vi "sort standard to sequence.vi"(8 "error in":errorcluster) -> (3 "output cluster":T1, 11 "cycle results cluster IN":T2)   [LabVIEW 2016]
doc: "Takes a sample type and sorts by sequence"
uses:
  controls/cycle results control.ctl
  controls/data control cluster.ctl
panel:
  out "Array":dbl[][][](array[numeric])
  out "error out":errorcluster
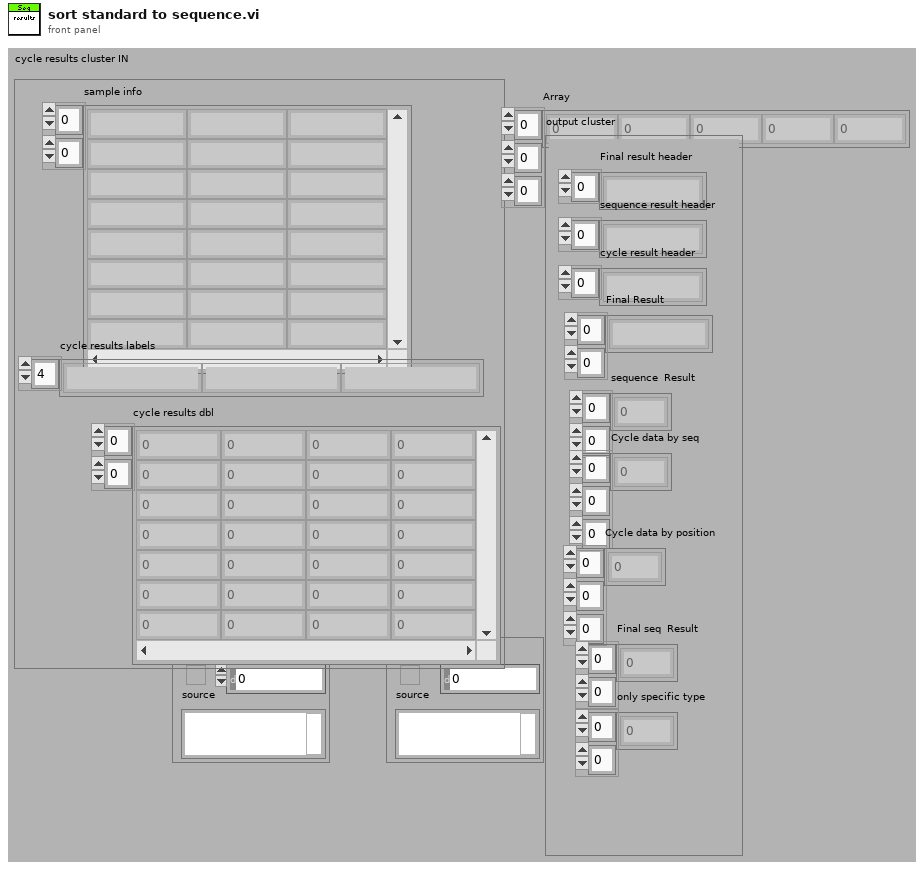
[diagram p1: front panel]
types:
  T1 = typedef "data control cluster.ctl" = cluster{"Final result header":string[], "sequence result header":string[], "cycle result header ":string[], "Final Result":string[][], "sequence  Result":dbl[][], "Cycle data by seq":dbl[][][], "Cycle data by position":dbl[][][], "Final seq  Result":dbl[][], "only specific type":dbl[][]}
  T2 = typedef "cycle results control.ctl" = cluster{"sample info":string[][], "cycle results labels":string[], "cycle results dbl":dbl[][]}
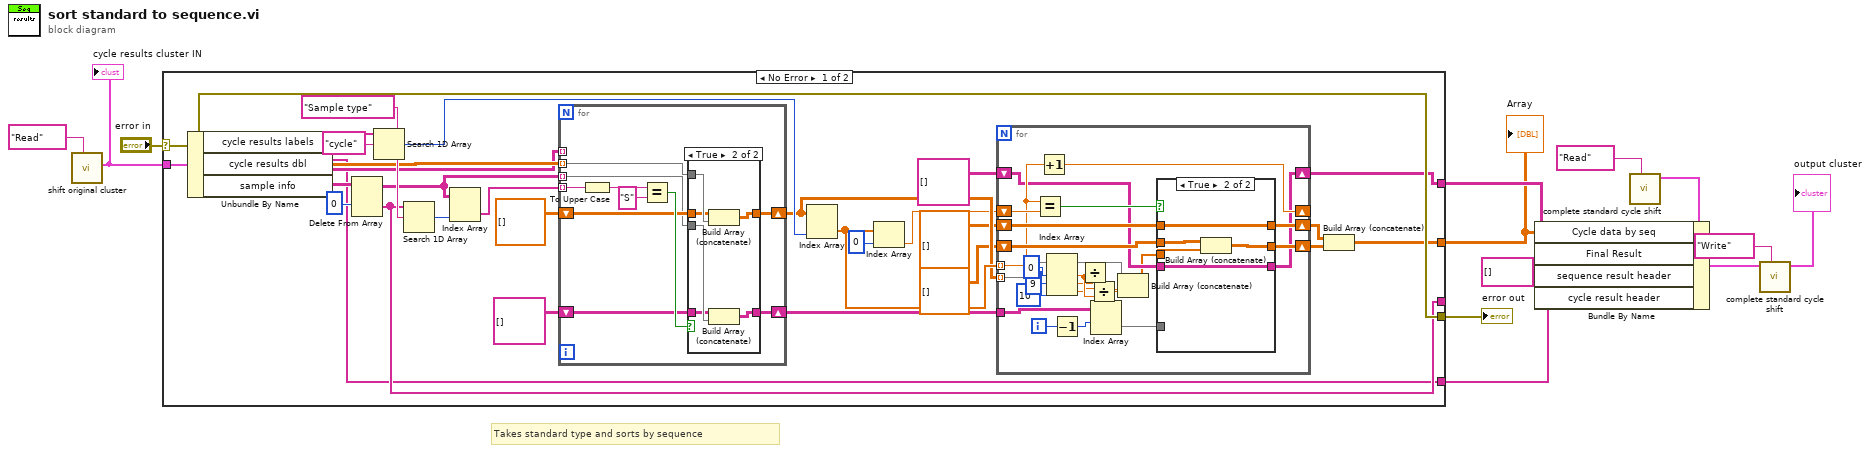
[diagram p0: block diagram]
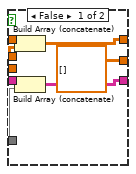
[diagram p2: hidden frame]
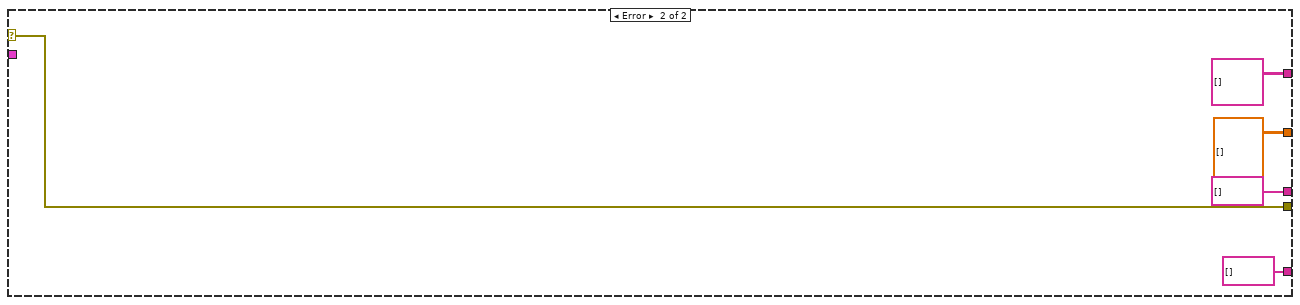
[diagram p4: hidden frame]
diagram:
  # "Takes standard type and sorts by sequence"
  n1 = call "shift original cluster.vi"("read write shift"="Read") -> ("cycle results cluster out"=w9:T2)  [unwired: 9 in, 1 out]
  "cycle results cluster IN" <- w9
  n2 = case shown="No Error" "error in" {
    selector: "error in" -> [w39 w98]
    tunnel: w9 -> [w38 _]
    tunnel: [w39 w98] -> w11
    tunnel: [w16 string[][] []] -> w5
    tunnel: [w15 string[] [] ("sample info")] -> _
    tunnel: [w14 dbl[][][] []] -> w4
    tunnel: [w13 string[] [] ("cycle results labels")] -> w1
    frame No Error {
      n3 = Unbundle By Name(w38) -> ("cycle results labels"=w13:string[], "cycle results dbl"=w33:dbl[][], "sample info"=w31:string[][])
      n4 = Delete From Array(array=w31, index (row)=0) -> (deleted portion=w15:string[], array with subset deleted=w30:string[][])  [unwired: 2 in]
      n5 = Search 1D Array(1D array=w13, element="cycle") -> (index of element=w27:i32)  [unwired: 1 in]
      n6 = Search 1D Array(1D array=w15, element="Sample type") -> (index of element=w35:i32)  [unwired: 1 in]
      n7 = Index Array(array=w30, index (col)=w35) -> (element=w34:string[])  [unwired: 1 in]
      n8 = for {
        tunnel: w31 -> [_] mode=indexing
        tunnel: w33 -> [w81] mode=indexing
        tunnel: w34 -> [w85] mode=indexing
        shift-right: [w80] -> w25
        shift-left: dbl[][] [] -> [w79]
        tunnel: w30 -> [w78] mode=indexing
        shift-right: [w77] -> w18
        shift-left: string[][] [] -> [w76]
        n9 = To Upper Case(1:w85) -> (0:w84:string)
        n10 = Equal?(x=w84, y="S") -> (x = y?=w82:bool)
        n11 = case shown="True" w82 {
          tunnel: w81 -> [_ w93]
          tunnel: [w87 w92] -> w80
          tunnel: w79 -> [w87 w91]
          tunnel: w78 -> [_ w90]
          tunnel: [w86 w88] -> w77
          tunnel: w76 -> [w86 w89]
          frame False {
          }
          frame True {
            n12 = Build Array (concatenate)(w91, w93) -> (w92:dbl[][])
            n13 = Build Array (concatenate)(w89, w90) -> (w88:string[][])
          }
        }
      }
      n14 = Index Array(array=w25, index (col)=w27) -> (element=w26:dbl[])  [unwired: 1 in]
      n15 = Index Array(array=w26, index=0) -> (element=w19:dbl)
      n16 = for {
        tunnel: w26 -> [w57] mode=indexing
        shift-right: [w56] -> _
        shift-left: w19 -> [w63]
        tunnel: w25 -> [w43] mode=indexing
        shift-right: [w62] -> w22
        shift-left: dbl[][] [] -> [w61]
        shift-right: [w60] -> w21
        shift-left: dbl[][][] [] -> [w59]
        tunnel: w18 -> [w55]
        shift-right: [w53] -> w16
        shift-left: string[][] [] -> [w51]
        i -> [w54]
        n17 = Equal?(x=w57, y=w63) -> (x = y?=w58:bool)
        n18 = Increment(x=w57) -> (x+1=w56:dbl)
        n19 = Index Array(array=w43, index #1=0 ("index"), index #2=9 ("index"), index #3=10 ("index")) -> (element #1=w46:dbl, element #2=w44:dbl, element #3=w45:dbl)
        n20 = Decrement(x=w54) -> (x-1=w50:i32)
        n21 = Divide(x=w44, y=w46) -> (x/y=w42:dbl)
        n22 = Divide(x=w45, y=w46) -> (x/y=w41:dbl)
        n23 = Index Array(array=w55, index (row)=w50) -> (element=w52:string[])  [unwired: 1 in]
        n24 = Build Array (concatenate)(w43, w42, w41) -> (w40:dbl[])
        n25 = case shown="True" w58 {
          tunnel: w40 -> [_ w75]
          tunnel: [dbl[][] [] w74] -> w62
          tunnel: w61 -> [w70 w73]
          tunnel: [w69 w72] -> w60
          tunnel: w59 -> [w68 w72]
          tunnel: [w64 w71] -> w53
          tunnel: w52 -> [w66 _]
          tunnel: w51 -> [w65 w71]
          frame False {
            n26 = Build Array (concatenate)(w68, w70) -> (w69:dbl[][][])
            n27 = Build Array (concatenate)(w65, w66) -> (w64:string[][])
          }
          frame True {
            n28 = Build Array (concatenate)(w73, w75) -> (w74:dbl[][])
          }
        }
      }
      n29 = Build Array (concatenate)(w21, w22) -> (w14:dbl[][][])
    }
    frame Error {
    }
  }
  "error out" <- w11
  "Array" <- w4
  n30 = call "complete standard cycle shift.vi"("read write shift"="Read") -> ("DATA CLUSTER out"=w6:T1)  [unwired: 9 in, 1 out]
  n31 = Bundle By Name(cluster=w6, "Cycle data by seq"=w4, "Final Result"=w5, "sequence result header"=string[] [], "cycle result header"=w1) -> (w3:T1)
  "output cluster" <- w3
  n32 = call "complete standard cycle shift.vi"("read write shift"="Write", "DATA CLUSTER in"=w3) -> ()  [unwired: 8 in, 2 out]
